vi "Write Reference VI Ref.vi"(10 "Reference VI Ref":refnum<vi>, 11 "Prototyper in":refnum<class "Prototyper.lvclass">) -> (3 "Prototyper out":refnum<class "Prototyper.lvclass">)   [LabVIEW 2020, in "Message Maker.lvlib" / "Prototyper.lvclass"]
uses:
  Prototyper.lvclass
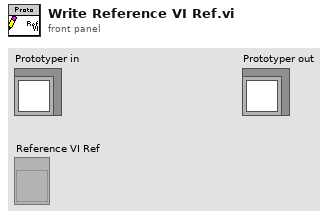
[diagram p1: front panel]
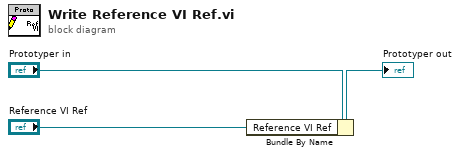
[diagram p0: block diagram]
diagram:
  n1 = Bundle By Name(cluster="Prototyper in", "Reference VI Ref"="Reference VI Ref") -> (→"Prototyper out":refnum<class "Prototyper.lvclass">)
